vi "CAL_FLOW_SENSOR.vi"(8 "error in (no error)":errorcluster, 11 "flow_slope_IN":dbl=51.35 format="%.2f") -> (0 "error out":errorcluster, 3 "flow_slope_OUT":dbl=51.35 format="%.2f")   [LabVIEW 2016]
uses:
  ad interface/Global_SIM_switch.vi
panel:
  out "Flow":dbl format="%.2f"
  in  "stop":bool
  in  "start":bool
  # "FLOW SENSOR CALIBRATION"
  # "Start Kpro flow. Allow the flow to equilibrate."
  # "After flow has equilibrated,  Press Start, simultaneously move Kpro effluent into graduated cylinder."
  # "Press Stop when 100 mL of water has been collected."
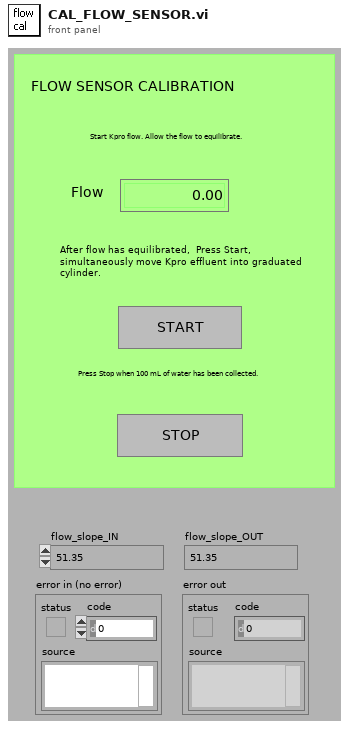
[diagram p1: front panel]
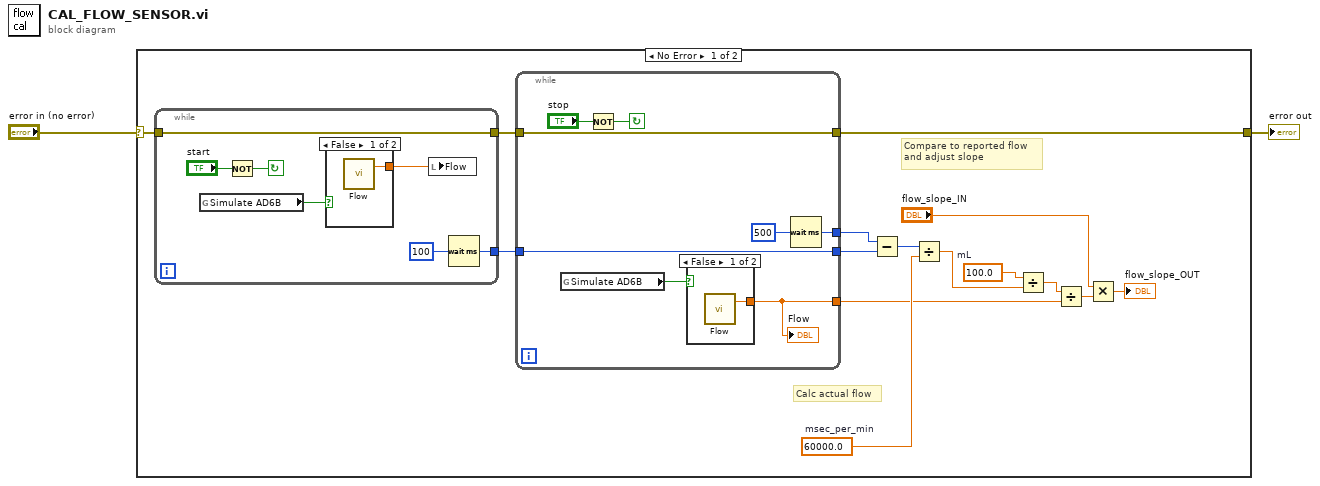
[diagram p0: block diagram]
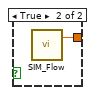
[diagram p2: hidden frame]
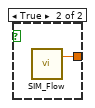
[diagram p3: hidden frame]
diagram:
  n1 = case shown="No Error" "error in (no error)" {
    selector: "error in (no error)" -> [w17 w37]
    tunnel: [w15 w37] -> w2
    frame No Error {
      w10 = 60000.0  # msec_per_min
      w11 = 100.0  # mL
      # "Compare to reported flow\nand adjust slope"
      # "Calc actual flow"
      n2 = while {
        tunnel: [w20] -> w16
        tunnel: w17 -> [w20]
        tunnel: [w21] -> w14
        stop <- w23 continue-if-true
        n3 = global read "Global_SIM_switch.vi" "Simulate AD6B"() -> (w19:bool)
        n4 = Not(x="start") -> (.not. x?=w23:bool)
        n5 = case shown="False" w19 {
          tunnel: [w25 w26] -> w18
          frame False {
            n6 = call "Flow.vi"() -> ("Flow (ml/min)"=w25:dbl)  [unwired: 3 in]
          }
          frame True {
            n7 = call "SIM_Flow.vi"() -> ("Flow (ml/min)"=w26:dbl)  [unwired: 3 in]
          }
        }
        n8 = local write "Flow"(w18) -> ()
        n9 = Wait (ms)(milliseconds to wait=u32 100) -> (millisecond timer value=w21:u32)
      }
      n10 = while {
        tunnel: [w27] -> w3
        tunnel: w14 -> [w28]
        tunnel: [w28] -> w12
        tunnel: w16 -> [w29]
        tunnel: [w29] -> w15
        tunnel: [w32] -> w13
        stop <- w34 continue-if-true
        n11 = global read "Global_SIM_switch.vi" "Simulate AD6B"() -> (w30:bool)
        n12 = Not(x="stop") -> (.not. x?=w34:bool)
        n13 = case shown="False" w30 {
          tunnel: [w35 w36] -> w27
          frame False {
            n14 = call "Flow.vi"() -> ("Flow (ml/min)"=w35:dbl)  [unwired: 3 in]
          }
          frame True {
            n15 = call "SIM_Flow.vi"() -> ("Flow (ml/min)"=w36:dbl)  [unwired: 3 in]
          }
        }
        "Flow" <- w27
        n16 = Wait (ms)(milliseconds to wait=u32 500) -> (millisecond timer value=w32:u32)
      }
      n17 = Subtract(x=w13, y=w12) -> (x-y=w9:u32)
      n18 = Divide(x=w9, y=w10) -> (x/y=w8:dbl)
      n19 = Divide(x=w11, y=w8) -> (x/y=w4:dbl)
      n20 = Divide(x=w4, y=w3) -> (x/y=w7:dbl)
      n21 = Multiply(x="flow_slope_IN", y=w7) -> (x*y=→"flow_slope_OUT":dbl)
    }
    frame Error {
    }
  }
  "error out" <- w2
